vi "Test_PublishUnnamed_PublicationIgnored_MediatorContinues.vi"(8 "error in (no error)":errorcluster, 11 "TestMediator In":refnum<class "TestMediationSemantics.lvclass">) -> (0 "error out":errorcluster, 3 "TestMediator Out":refnum<class "TestMediationSemantics.lvclass">)   [LabVIEW 2017, in "TestMediationSemantics.lvclass"]
uses:
  TestMediationSemantics.lvclass
  gpm_packages/@cs/mva-core/Source/Mediator/Mediator/Mediator.lvclass
  <vilib>/ActorFramework/Actor/Actor.lvclass
  gpm_packages/@cs/mva-core/Source/IMediator/IMediator Messages/Publish Msg/Publish Msg.lvclass
  <vilib>/ActorFramework/Stop Msg/Stop Msg.lvclass
  gpm_packages/@cs/mva-core/Source/IMediator/PublishRequest/PublishRequest.lvclass
  gpm_packages/@cs/transport/Source/Concrete/QueueTransport/QueueTransport.lvclass
  gpm_packages/@cs/mva-core/Source/IMediator/IMediator Messages/Lock Publication Msg/Lock Publication Msg.lvclass
  <vilib>/addons/_JKI Toolkits/VI Tester/TestCase.llb/TestCase.lvclass
  C:/Program Files (x86)/National Instruments/LabVIEW 2017/vi.lib/addons/_JKI Toolkits/VI Tester/TestCase.llb/TestCase.lvclass
  C:/Git/mva-framework/gpm_packages/@cs/mva-core/Source/IMediator/IMediator/IMediator.lvclass
  C:/Program Files (x86)/National Instruments/LabVIEW 2017/vi.lib/ActorFramework/Actor/Actor.lvclass
  C:/Git/mva-framework/gpm_packages/@cs/transport/Source/ITransport/ITransport.lvclass
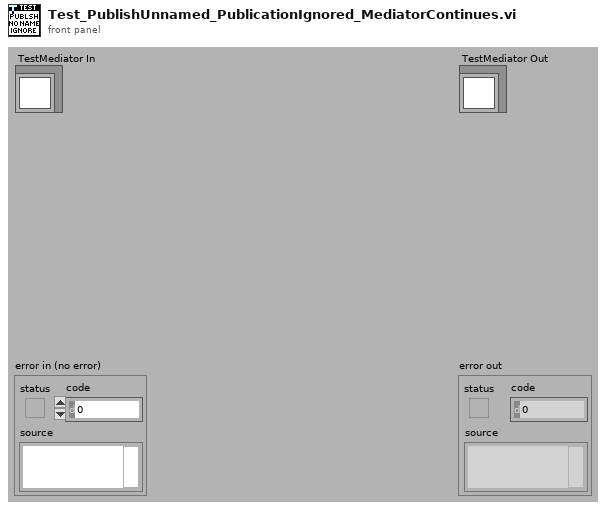
[diagram p1: front panel]
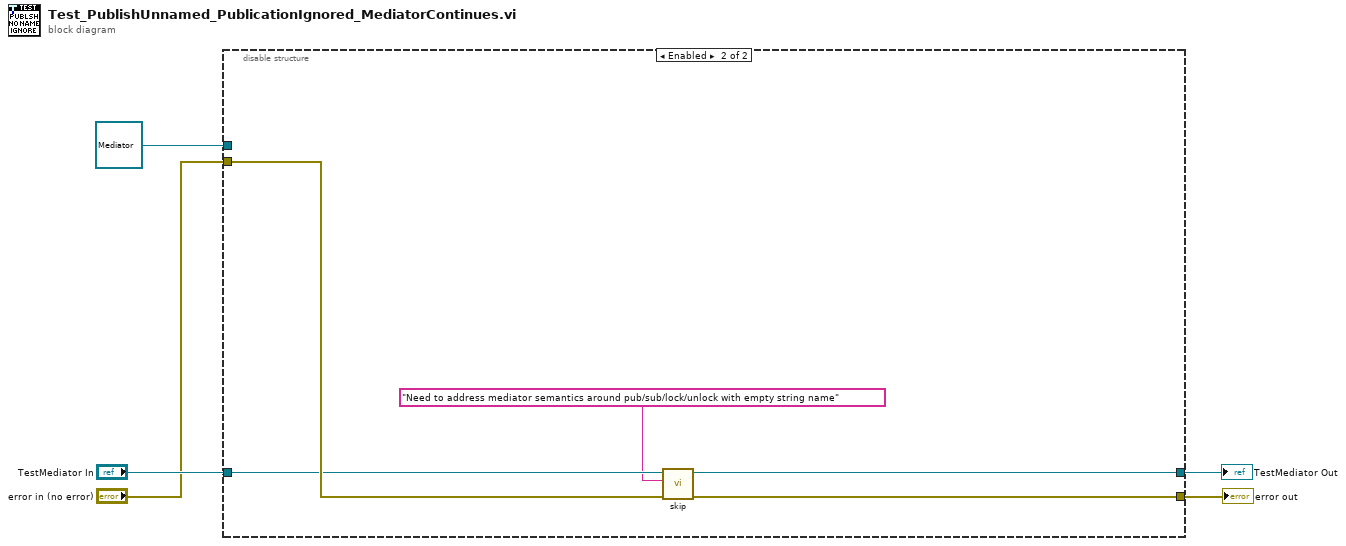
[diagram p0: block diagram]
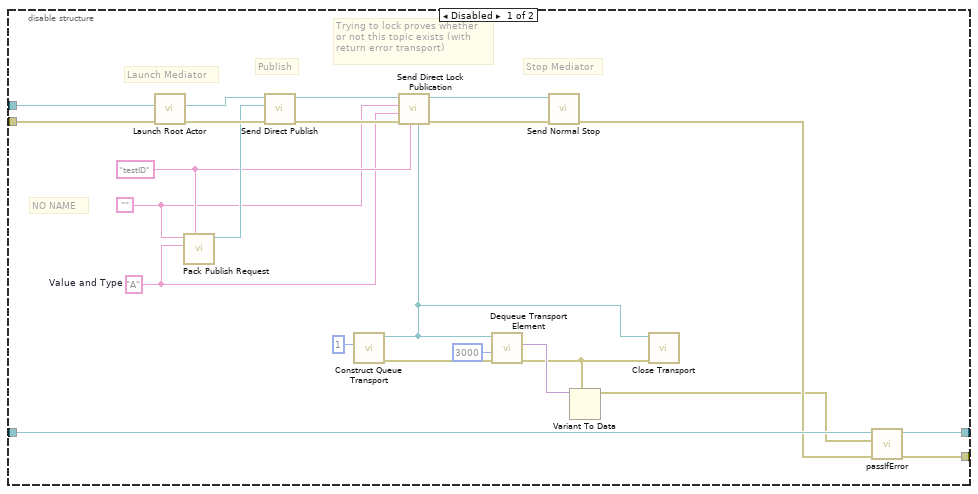
[diagram p2: hidden frame]
diagram:
  n1 = disable-structure shown="Enabled" {
    disable-tunnel: [w28 w32] -> w5
    disable-tunnel: "TestMediator In" -> [w27 w30]
    disable-tunnel: [w26 w31] -> w3
    disable-tunnel: refnum<class "Mediator.lvclass"> refnum ("Mediator.lvlib:Mediator.lvclass") -> [w25 _]
    disable-tunnel: "error in (no error)" -> [w9 w33]
    frame Disabled {
      w13 = "testID" ("Publisher ID")
      w11 = "" ("Datum Name")
      w12 = "A"  # Value and Type
      # "NO NAME"
      # "Launch Mediator"
      # "Stop Mediator"
      # "Trying to lock proves whether\nor not this topic exists (with\nreturn error transport)"
      # "Publish"
      n2 = call <vilib>:"Launch Root Actor.vi"("error in (no error)"=w9, "Actor"=w25) -> ("error out"=w20:errorcluster, "Actor's Enqueuer"=w24:refnum<class "Message Enqueuer.lvclass">)  [unwired: 8 in]
      n3 = call "Pack Publish Request.vi"("Publisher ID"=w13, "Datum Name"=w12, "PublishRequest In"=w11) -> ("PublishRequest Out"=w19:refnum<class "PublishRequest.lvclass">)  [unwired: 7 in, 1 out]
      n4 = call "Send Direct Publish.vi"("error in (no error)"=w20, "PublishRequest"=w19, "Mediator Enqueuer"=w24) -> ("error out"=w16:errorcluster, "Mediator Enqueuer out"=w18:refnum<class "Message Enqueuer.lvclass">)  [unwired: 7 in]
      n5 = call "Construct Queue Transport.vi"("Max Queue Size (-1)"=1) -> ("error out"=w7:errorcluster, "QueueTransport"=w14:refnum<class "QueueTransport.lvclass">)  [unwired: 9 in]
      n6 = call "Send Direct Lock Publication.vi"("Return Error Transport"=w14, "Publisher ID"=w13, "error in (no error)"=w16, "Datum Type"=w12, "Datum Name"=w11, "Mediator Enqeuer"=w18) -> ("error out"=w15:errorcluster, "Mediator Enqueuer out"=w17:refnum<class "Message Enqueuer.lvclass">)  [unwired: 4 in]
      n7 = call "Dequeue Transport Element.vi"("error in (no error)"=w7, "Timeout In ms (-1)"=3000, "QueueTransport"=w14) -> ("error out"=w10:errorcluster, "Data"=w21:variant)  [unwired: 5 in, 2 out]
      n8 = call <vilib>:"Send Normal Stop.vi"("error in (no error)"=w15, "Message Enqueuer"=w17) -> ("error out"=w8:errorcluster)  [unwired: 9 in]
      n9 = Variant To Data(type=w10, Variant=w21) -> (data=w6:errorcluster)  [unwired: 1 in, 1 out]
      n10 = call-dynamic "Close Transport.vi"("error in (no error)"=w10, "QueueTransport"=w14) -> ()  [unwired: 9 in, 1 out]
      n11 = call-dynamic "passIfError.vi"("error in (no error)"=w8, "error"=w6, "TestCase in"=w27) -> ("error out"=w28:errorcluster, "TestCase out"=w26:refnum<class "TestMediationSemantics.lvclass">)  [unwired: 7 in]
    }
    frame Enabled {
      n12 = call <vilib>:"skip.vi"("error in (no error)"=w33, "skipMessage"="Need to address mediator semantics around pub/sub/lock/unlock with empty string name", "TestCase in"=w30) -> ("error out"=w32:errorcluster, "TestCase out"=w31:refnum<class "TestMediationSemantics.lvclass">)  [unwired: 7 in]
    }
  }
  "error out" <- w5
  "TestMediator Out" <- w3
